vi "iterate_variables.vi"(8 "error in (no error)":errorcluster, 9 "Variable Settings Refnum":refnum<vi>, 10 "Current Iteration":i32, 11 "ExperimentVariables in":refnum<class "ExperimentVariables.lvclass">) -> (0 "error out":errorcluster, 3 "ExperimentVariables out":refnum<class "ExperimentVariables.lvclass">)   [LabVIEW 2013, in "ExperimentVariables.lvclass"]
uses:
  ExperimentVariables.lvclass
  Variable_Settings.ctl
  ExperimentVariables.lvclass/ExperimentVariables.ctl
panel:
  # "Parameters will be evaluated once at the beginning of the experiment from top to bottom, \nso any parameter may depend on all those above it.\nVariables will be evaluated each iteration.\nParameters and Variables may be used in various other experiment settings, as noted.\nSee LabView Help -> Formula Node and Expression Node Functions for a list of available functions."
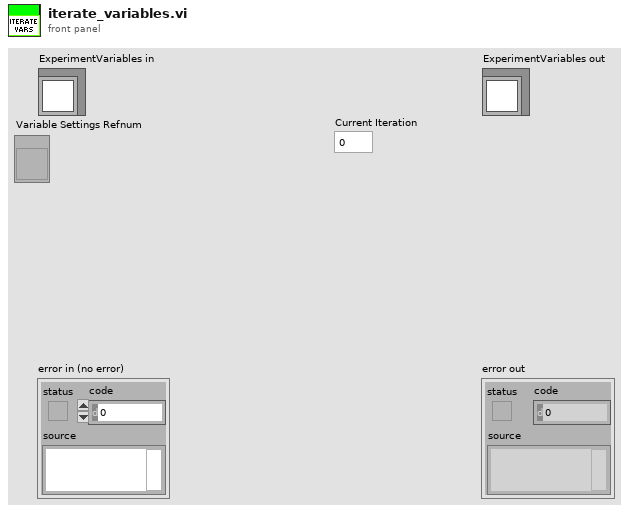
[diagram p1: front panel]
types:
  T1 = typedef "ExperimentVariables.lvclass/Variable_Settings.ctl" = cluster{"Measurements per Iteration":i32, "Local Data Path":path, "Experiment description suffix for filename (no spaces please)":string, "Network Data Path":path, "Copy data to network":bool, "Measurement Timeout (ms)":u32, "Independent Variables":cluster{"Description":string, "Name (a,a0...a9)":string, "min":dbl, "max":dbl, "# steps":u32}[], "Dependent Variables":cluster{"Description":string, "Name (a,a0...a9)":string, "Equation":string, "Result":dbl}[], "Run Test Mode":bool}
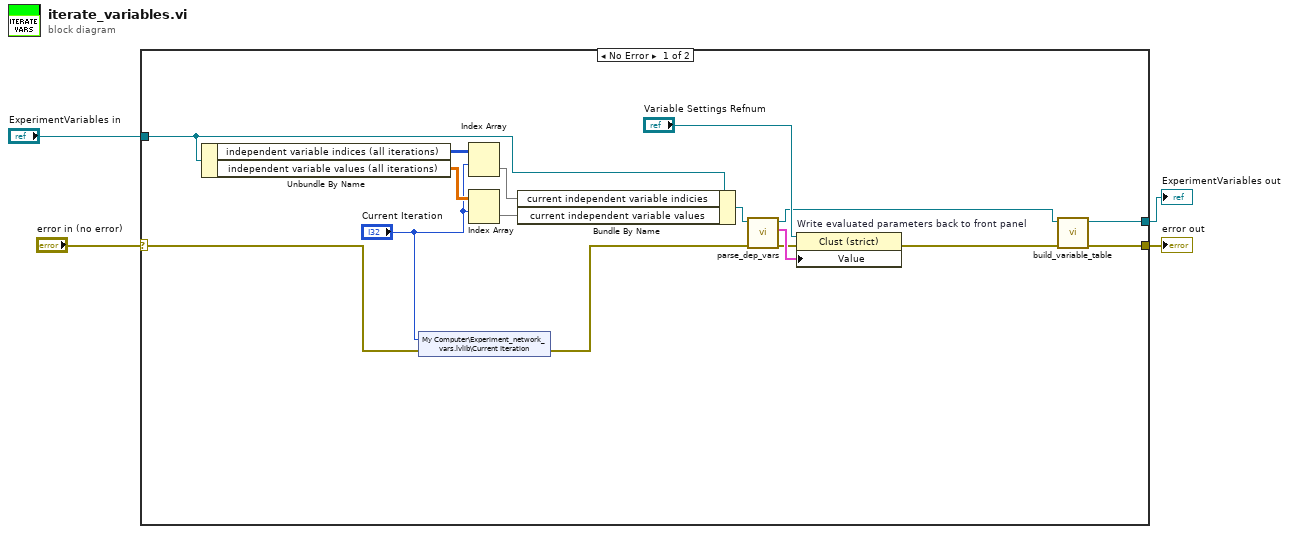
[diagram p0: block diagram]
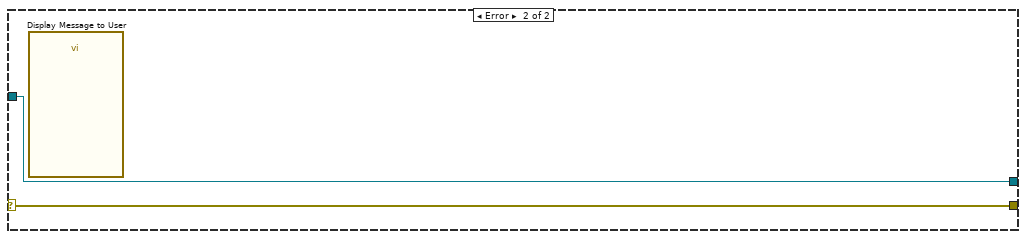
[diagram p2: hidden frame]
diagram:
  n1 = case shown="No Error" "error in (no error)" {
    selector: "error in (no error)" -> [w8 w22]
    tunnel: [w6 w22] -> w3
    tunnel: [w5 w21] -> w1
    tunnel: "ExperimentVariables in" -> [w18 w21]
    frame No Error {
      n2 = Unbundle By Name(w18) -> ("independent variable indices (all iterations)"=w20:i32[][], "independent variable values (all iterations)"=w19:dbl[][])
      n3 = shared-variable "My Computer\\Experiment_network_vars.lvlib\\Current Iteration"("Current Iteration", error in=w8) -> (error out=w7:errorcluster)
      n4 = Index Array(array=w20, index (row)="Current Iteration") -> (element=w17:i32[])  [unwired: 1 in]
      n5 = Index Array(array=w19, index (row)="Current Iteration") -> (element=w16:dbl[])  [unwired: 1 in]
      n6 = Bundle By Name(cluster=w18, "current independent variable indicies"=w17, "current independent variable values"=w16) -> (w11:refnum<class "ExperimentVariables.lvclass">)
      n7 = call-dynamic "parse_dep_vars.vi"("error in (no error)"=w7, "ExperimentVariables in"=w11) -> ("error out"=w13:errorcluster, "Variable Settings (out)"=w15:T1, "ExperimentVariables out"=w10:refnum<class "ExperimentVariables.lvclass">)  [unwired: 7 in]
      n8 = property on="Write evaluated parameters back to front panel" class="Clust (strict)"(reference="Variable Settings Refnum", error in=w13, "Value"=w15) -> (error out=w12:errorcluster)  [unwired: 1 out]
      n9 = call-dynamic "build_variable_table.vi"("error in (no error)"=w12, "ExperimentVariables in"=w10) -> ("error out"=w6:errorcluster, "ExperimentVariables out"=w5:refnum<class "ExperimentVariables.lvclass">)  [unwired: 8 in]
    }
    frame Error {
      n10 = call "Display Message to User"() -> ()  [unwired: 10 in, 2 out]
    }
  }
  "error out" <- w3
  "ExperimentVariables out" <- w1
